vi "Close.vi"(8 "error in (no error)":errorcluster, 11 "Task Base in":refnum<class "Task Base.lvclass">) -> (0 "error out":errorcluster, 3 "Task Base out":refnum<class "Task Base.lvclass">)   [LabVIEW 2023, in "HAL GOOP4.lvlib" / "Task Base.lvclass"]
uses:
  Task Base.lvclass
  Task Base.lvclass/Task Base.ctl
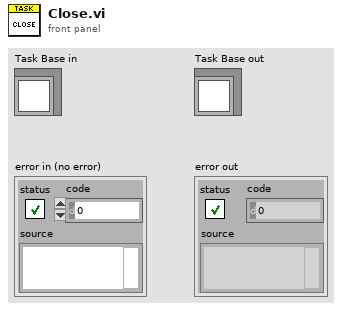
[diagram p1: front panel]
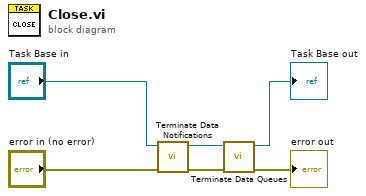
[diagram p0: block diagram]
diagram:
  n1 = call-dynamic "Terminate Data Notifications.vi"("error in (no error)"="error in (no error)", "Task Base in"="Task Base in") -> ("error out"=w5:errorcluster, "Task Base out"=w2:refnum<class "Task Base.lvclass">)  [unwired: 8 in]
  n2 = call-dynamic "Terminate Data Queues.vi"("error in (no error)"=w5, "Task Base in"=w2) -> ("error out"=→"error out":errorcluster, "Task Base out"=→"Task Base out":refnum<class "Task Base.lvclass">)  [unwired: 8 in]
